vi "Utility - Exit Program if executable.vi"(8 "error in (no error)":errorcluster, 10 "Force LabVIEW Exit?":bool) -> (0 "error out":errorcluster)   [LabVIEW 2014]
panel:
  # "INPUTS"
  # "OUTPUTS"
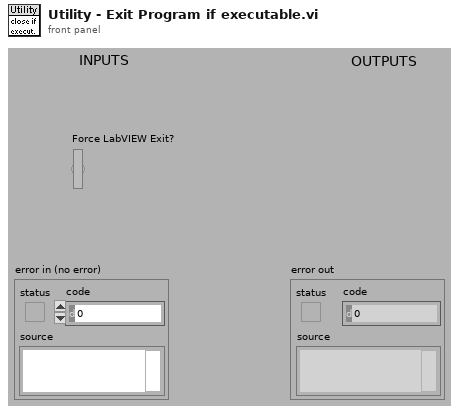
[diagram p1: front panel]
types:
  T1 = enum32{"invalid app kind", "Development System", "Run Time System", "Student Edition", "Embedded LabVIEW", "Evaluation", "Custom"}
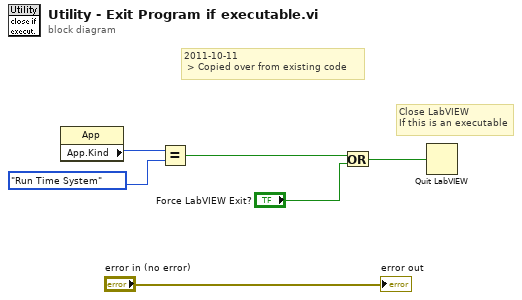
[diagram p0: block diagram]
diagram:
  # "2011-10-11\n > Copied over from existing code"
  # "Close LabVIEW\nIf this is an executable"
  n1 = property class="App"() -> ("App.Kind"=w3:T1)  [unwired: 2 in, 2 out]
  n2 = Equal?(x=w3, y=T1."Run Time System" ("Application:Kind")) -> (x = y?=w1:bool)
  n3 = Or(x=w1, y="Force LabVIEW Exit?") -> (x .or. y?=w5:bool)
  n4 = Quit LabVIEW(quit? (T)=w5) -> ()
  "error out" <- "error in (no error)"
